vi "Points2PolynomialInterpolation.vi"(9 "Alpha Value":dbl, 10 "Velocities":cluster{"Initial ":dbl, "Final":dbl}, 11 "Positions":cluster{"Initial ":dbl, "Final":dbl}) -> (3 "Polynomial Coefficients (final = leading)":dbl[](array[numeric]))   [LabVIEW 2016]
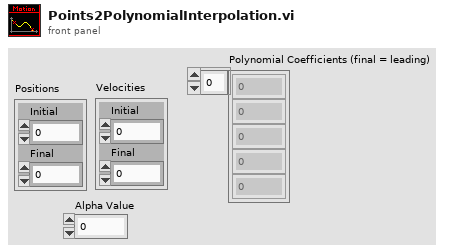
[diagram p1: front panel]
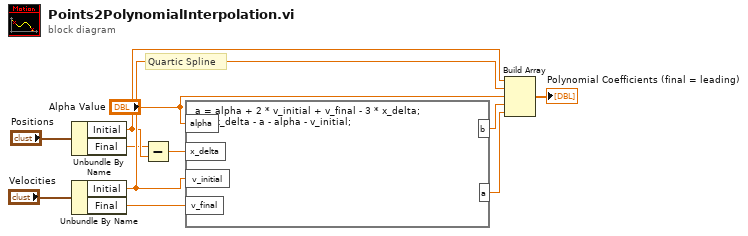
[diagram p0: block diagram]
diagram:
  # "Quartic Spline"
  n1 = Unbundle By Name("Positions") -> ("Initial"=w2:dbl, "Final"=w1:dbl)
  n2 = Unbundle By Name("Velocities") -> ("Initial"=w7:dbl, "Final"=w8:dbl)
  n3 = Subtract(x=w1, y=w2) -> (x-y=w9:dbl)
  n4 = formula code="a = alpha + 2 * v_initial + v_final - 3 * x_delta;\nb = x_delta - a - alpha - v_initial;"("alpha"="Alpha Value", "x_delta"=w9, "v_initial"=w7, "v_final"=w8) -> ("a"=w4:dbl, "b"=w5:dbl)
  n5 = Build Array(w2, w7, "Alpha Value", w5, w4) -> (→"Polynomial Coefficients (final = leading)":dbl[])
